vi "Test.vi"(8 "error in (no error)":errorcluster, 11 "Concrete Test Step in":refnum<class "Concrete Test Step.lvclass">) -> (0 "error out":errorcluster, 2 "Pass?":bool, 3 "Concrete Test Step out":refnum<class "Concrete Test Step.lvclass">)   [LabVIEW 2020, in "Concrete Test Step.lvclass"]
uses:
  Concrete Test Step.lvclass
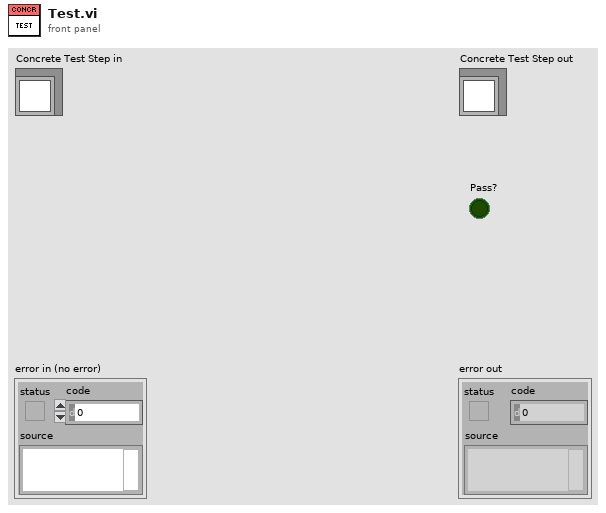
[diagram p1: front panel]
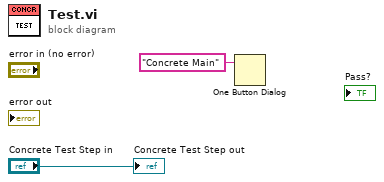
[diagram p0: block diagram]
diagram:
  n1 = One Button Dialog(message="Concrete Main") -> ()  [unwired: 1 in, 1 out]
  "Concrete Test Step out" <- "Concrete Test Step in"
